vi "研华USBIO读写功能函数集.vi"(8 "error in (no error)":errorcluster caption="错误输入（无错误）", 9 "IO输出":T1, 11 "选项":T3) -> (0 "error out":errorcluster caption="错误输出", 1 "结果":bool, 2 "IO输入":T2, 3 "Read Data":bool[](array[boolean]), 4 "IO输出":T1)   [LabVIEW 2014]
uses:
  IOinput.ctl
  IOoutput.ctl
  <userlib>/DAQNavi Polymorphic VI/create/DAQNavi Create Channel(DI-Digital Input).vi
  <userlib>/DAQNavi Polymorphic VI/create/DAQNavi Create Channel(DO-Digital Output).vi
  <userlib>/DAQNavi Polymorphic VI/read/DAQNavi Read (Digital 1D U8 NChan 1Samp).vi
  <userlib>/DAQNavi Polymorphic VI/write/DAQNavi Write (Digtial 1D U8 NChan 1Samp).vi
panel:
  out "Read data":u8[](array[numeric])
  out "physical channels output":string="DemoDevice,BID#0/port0:1" caption="property value"
  out "physical channels input":string="DemoDevice,BID#0/port0:1" caption="property value"
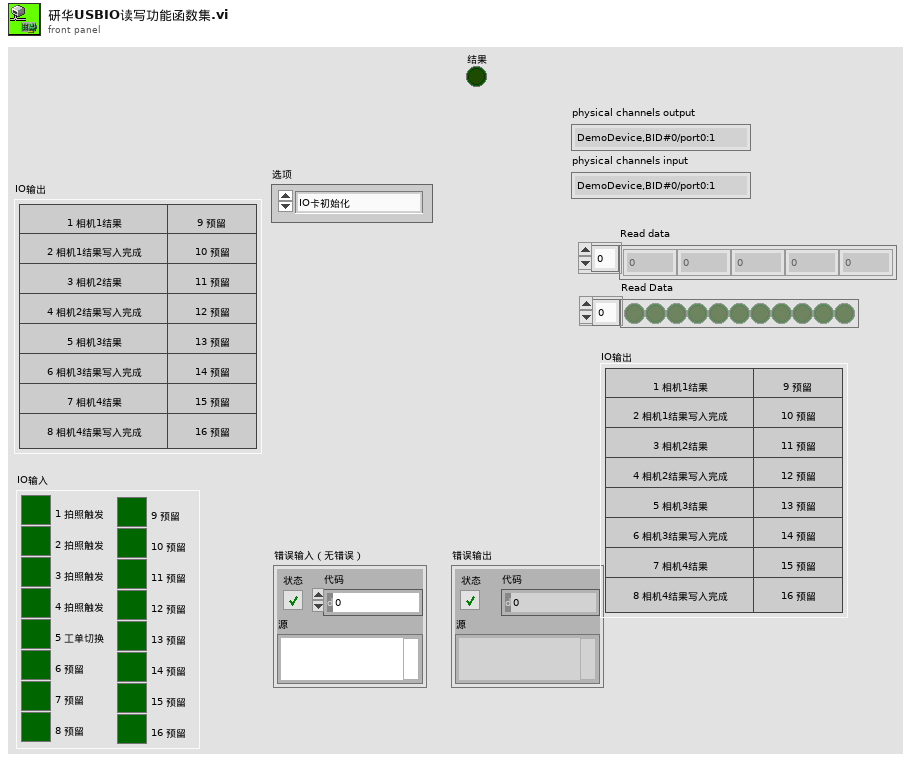
[diagram p1: front panel]
types:
  T1 = typedef "IOoutput.ctl" = cluster{"1 相机1结果":bool, "2 相机1结果写入完成":bool, "3 相机2结果":bool, "4 相机2结果写入完成":bool, "5 相机3结果":bool, "6 相机3结果写入完成":bool, "7 相机4结果":bool, "8 相机4结果写入完成":bool, "9预留":bool, "10预留":bool, "11预留":bool, "12预留":bool, "13预留":bool, "14预留":bool, "15预留":bool, "16预留":bool}
  T2 = typedef "IOinput.ctl" = cluster{"1 拍照触发":bool, "2 拍照触发":bool, "3 拍照触发":bool, "4 拍照触发":bool, "5 工单切换":bool, "6 预留":bool, "7 预留":bool, "8 预留":bool, "9 预留":bool, "10 预留":bool, "11 预留":bool, "12 预留":bool, "13 预留":bool, "14 预留":bool, "15 预留":bool, "16 预留":bool}
  T3 = typedef "研华USBIO功能函数集Action.ctl" = enum16{"IO卡初始化", "读取信号", "写入信号", "GetInfo", "清除目标"}
  T4 = cluster{"Write Data[0]":bool, "Write Data[1]":bool, "Write Data[2]":bool, "Write Data[3]":bool, "Write Data[4]":bool, "Write Data[5]":bool, "Write Data[6]":bool, "Write Data[7]":bool, "Write Data[8]":bool, "Write Data[9]":bool, "Write Data[10]":bool, "Write Data[11]":bool, "Write Data[12]":bool, "Write Data[13]":bool, "Write Data[14]":bool, "Write Data[15]":bool}
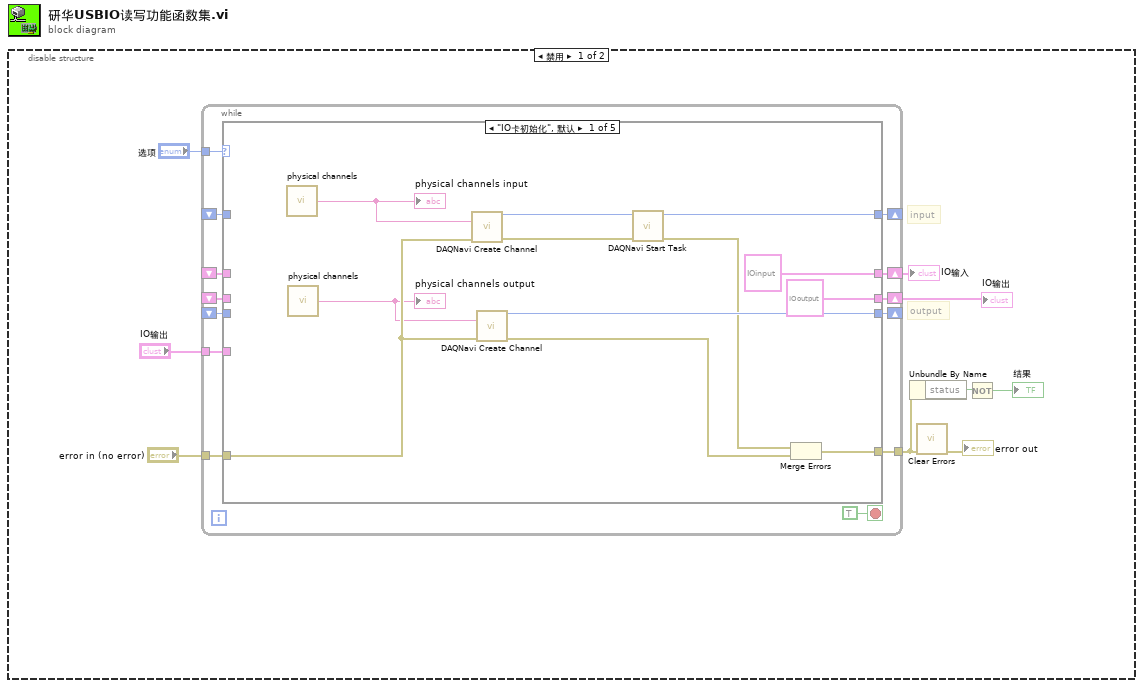
[diagram p0: block diagram]
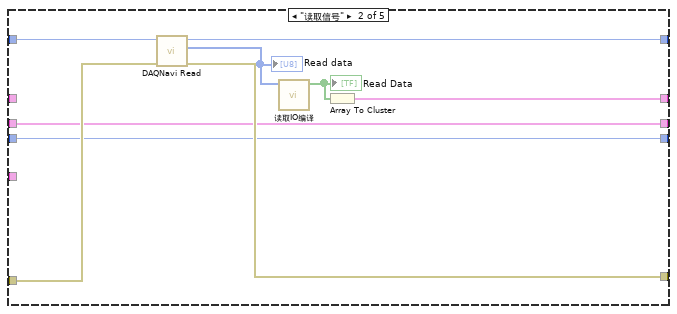
[diagram p2: hidden frame]
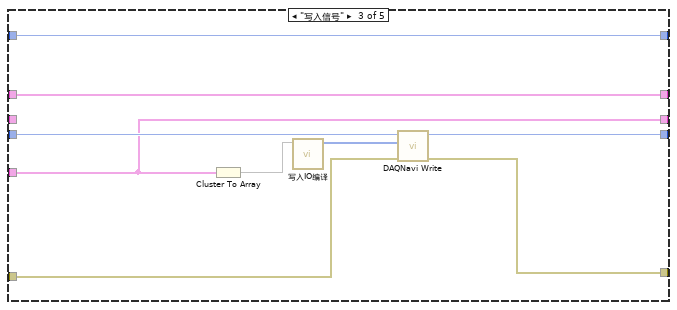
[diagram p3: hidden frame]
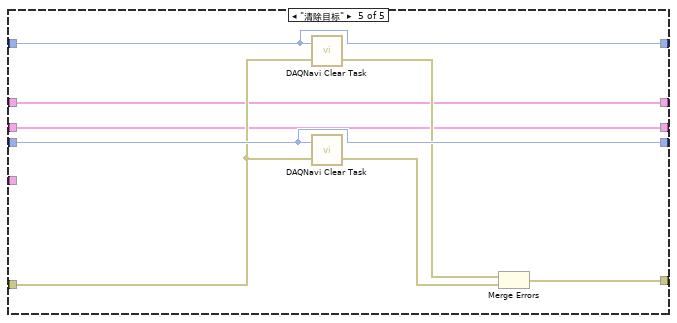
[diagram p5: hidden frame]
diagram:
  n1 = disable-structure shown="禁用" {
    frame Disabled {
      # "output"
      # "input"
      n2 = while {
        tunnel: "选项" -> [w21]
        shift-right: [w19] -> _
        shift-left: _ -> [w16]
        shift-right: [w20] -> _
        shift-left: _ -> [w15]
        tunnel: [w18] -> w3
        tunnel: "error in (no error)" -> [w17]
        shift-right: [w14] -> w7
        shift-left: _ -> [w13]
        shift-right: [w12] -> w5
        shift-left: _ -> [w11]
        tunnel: "IO输出" -> [w10]
        stop <- TRUE stop-if-true
        n3 = case shown="\"IO卡初始化\", 默认" w21 {
          tunnel: [w33 w39 w50 w56 w64] -> w20
          tunnel: [w31 w42 w52 w57 w65] -> w19
          tunnel: [w27 w40 w48 w54 w60] -> w18
          tunnel: w17 -> [w26 w41 w49 w54 w63]
          tunnel: w16 -> [_ w43 w52 w57 w65]
          tunnel: w15 -> [_ w39 w51 w56 w64]
          tunnel: [T2 {"1 拍照触发"=FALSE, "2 拍照触发"=FALSE, "3 拍照触发"=FALSE, "4 拍照触发"=FALSE, "5 工单切换"=FALSE, "6 预留"=FALSE, "7 预留"=FALSE, "8 预留"=FALSE, "9 预留"=FALSE, "10 预留"=FALSE, "11 预留"=FALSE, "12 预留"=FALSE, "13 预留"=FALSE, "14 预留"=FALSE, "15 预留"=FALSE, "16 预留"=FALSE} ("IO输入") w36 w45 w55 w59] -> w14
          tunnel: w13 -> [_ _ w45 w55 w59]
          tunnel: [T1 {"1 相机1结果"=FALSE, "2 相机1结果写入完成"=FALSE, "3 相机2结果"=FALSE, "4 相机2结果写入完成"=FALSE, "5 相机3结果"=FALSE, "6 相机3结果写入完成"=FALSE, "7 相机4结果"=FALSE, "8 相机4结果写入完成"=FALSE, "9预留"=FALSE, "10预留"=FALSE, "11预留"=FALSE, "12预留"=FALSE, "13预留"=FALSE, "14预留"=FALSE, "15预留"=FALSE, "16预留"=FALSE} ("IO输出") w35 w44 w53 w58] -> w12
          tunnel: w11 -> [_ w35 _ w53 w58]
          tunnel: w10 -> [_ _ w44 _ _]
          frame "IO卡初始化", Default {
            n4 = call "physical channels"() -> ("property value"=w34:string)  [unwired: 1 out]
            "physical channels input" <- w34
            n5 = call "physical channels"() -> ("property value"=w25:string)  [unwired: 1 out]
            "physical channels output" <- w25
            n6 = call-poly <userlib>:"DAQNavi Create Channel.vi"("physical channels"=w34, "error in (no error)"=w26) -> ("task out"=w32:i32, "error out"=w30:errorcluster)  [unwired: 3 in, 9 out]
            n7 = call-poly <userlib>:"DAQNavi Create Channel.vi"("physical channels"=w25, "error in (no error)"=w26) -> ("task out"=w33:i32, "error out"=w29:errorcluster)  [unwired: 3 in, 9 out]
            n8 = call <userlib>:"DAQNavi Start Task.vi"("error in (no error)"=w30, "task in"=w32) -> ("error out"=w28:errorcluster, "task out"=w31:i32)  [unwired: 8 out]
            n9 = Merge Errors(w28, w29) -> (w27:errorcluster)
          }
          frame "读取信号" {
            n10 = call-poly <userlib>:"DAQNavi Read.vi"("error in (no error)"=w41, "task in"=w43) -> ("error out"=w40:errorcluster, "data"=w38:u8[], "task out"=w42:i32)  [unwired: 2 in, 5 out]
            "Read data" <- w38
            n11 = call "读取IO编译.vi"("Read data"=w38) -> ("Write Data"=w37:bool[])  [unwired: 10 in]
            "Read Data" <- w37
            n12 = Array To Cluster(array=w37) -> (cluster=w36:T4)
          }
          frame "写入信号" {
            n13 = Cluster To Array(cluster=w44) -> (array=w46:bool[])
            n14 = call "写入IO编译.vi"("Write Data"=w46) -> ("数据"=w47:u32[])  [unwired: 10 in]
            n15 = call-poly <userlib>:"DAQNavi Write.vi"("error in (no error)"=w49, "data"=w47, "task in"=w51) -> ("error out"=w48:errorcluster, "task out"=w50:i32)  [unwired: 1 in, 6 out]
          }
          frame "GetInfo" {
          }
          frame "清除目标" {
            n16 = call <userlib>:"DAQNavi Clear Task.vi"("error in (no error)"=w63, "task in"=w65) -> ("error out"=w62:errorcluster)  [unwired: 1 out]
            n17 = call <userlib>:"DAQNavi Clear Task.vi"("error in (no error)"=w63, "task in"=w64) -> ("error out"=w61:errorcluster)  [unwired: 1 out]
            n18 = Merge Errors(w62, w61) -> (w60:errorcluster)
          }
        }
      }
      "IO输入" <- w7
      "IO输出" <- w5
      n19 = Unbundle By Name(w3) -> ("status"=w2:bool)
      n20 = call <vilib>:"Clear Errors.vi"("error in (no error)"=w3) -> ("error out"=→"error out":errorcluster)  [unwired: 5 in, 1 out]
      n21 = Not(x=w2) -> (.not. x?=→"结果":bool)
    }
    frame Enabled {
    }
  }
